vi "WaveGenerator_Sample_Program_NoDDL.vi"(0 "System no.":i32=1 min=1 step=1, 1 "Stop refnum":refnum<vi>, 2 "Affected axis":string="1", 3 "Selection":T1, 5 "error in":errorcluster, 6 "Sine Parameters:":T3={"Xo (Start)"=0, "SIN_P Parameters"={"C"=200.0, "A"=10.0, "O"=0.0}, "N (Length)"=500, "Append? (&)"=FALSE} {"N (Length)" min=0 max=1000 step=1; "SIN_P Parameters"."O" format="%.6f"; "SIN_P Parameters"."A" format="%.6f"; "SIN_P Parameters"."C" format="%.6f"}, 7 "Ramp Parameters:":T2={"Xo (Start)"=0, "RAMP Parameters"={"C"=200.0, "J"=0.0, "A"=8.0, "O"=0.0}, "N (Length)"=500, "Append? (&)"=FALSE} {"N (Length)" min=0 max=1000 step=1; "RAMP Parameters"."O" format="%.6f"; "RAMP Parameters"."A" format="%.6f"; "RAMP Parameters"."J" format="%.6f"; "RAMP Parameters"."C" format="%.6f"}, 8 "Start position":dbl format="%.6f") -> (14 "Waveform":dbl[][](graph) caption="Graph showing the commanded (green) and measured (white) waveform.", 19 "Error out":errorcluster)   [LabVIEW 2014, in "PiFOC.lvlib"]
doc: "This VI demonstrates how to use the wave generator command VIs. It first moves the affected axis to a given start position. Then it runs in a loop, giving the user the options to write sine wave curve segments or ramps into the controllers wave buffer. Wave storage data points are limited to 1000 points to keep transfer times low. The segment length of one waveform - which normally defines the frequency - is predefined as 500 points in this example. Depending on the value of Append? (&), either the old buffer data is overwritten or the new wave will be appended to memory. Please take into account that you can append at most two waveforms since buffer size is limited to 1000 points as mentioned above. \n\nAdjust the following controls to modify the shape of the waveforms.\nN (Length): Waveform (i.e. the points to be modified) goes from 1 to Length. Datapoints from Length to 500 are filled with value of last wave point.\nXo (Start): Position where the first point of the waveform is located. \nC: Center point of the wave. If C = Length/2 then the wave is symmetrical.\nA: Amplitude of the waveform. F(x) = A*sin(x) + O\nO: Offset of the waveform. F(x) = A*sin(x) + O\nJ: Jerk. Means curvature in the transition to or from standstill.\n\nYou have to stop generator output prior to restarting it with a different parameter set. The Start Gen. and Stop Gen. buttons will enable or disable the wave generator output by sending \"WGO 0\" or \"WGO 1\" for the affected axis. The red Stop button stops the wave generator output on the specified axis and finishes the loop. Please respect the delays that occur while the controller is processing your commands. This is indicated by the \"Busy?\" indicator. See manual for further details. \n\nIn case of an error a button Clear Error will appear and the control buttons above will be disabled. Pressing this button will clear the error status and enable the control buttons again.\n\nSee User Manual for details about the use of the wave generator.\n\nRun XXXX_Configuration_Setup (with XXXX being the product number of your PI controller) prior to running this VI.\n\nValid for: E-709"
uses:
  PiFOC.lvlib
panel:
  in  "Wave Table":string="1"
  out "Gen. running?":bool
  in  "Clear Error":bool
  out "Busy?":bool
  out "Controller error":bool
  in  "Stop":bool
  # "Wave generator sample program without DDL functionality"
  # "This VI demonstrates how to use the wave generator command VIs. It first moves the affected axis to a given start position. Then it runs in a loop, giving the\nuser the options to write sine wave curve segments or ramps into the controllers wave buffer. Wave storage data points are limited to 1000 points\nto keep transfer times low. The segment length of one waveform is predefined as 500 points in this example. Depending on the value of Append? (&), either\nthe old buffer data is overwritten or the new wave will be appended to memory. You have to stop generator output prior to restarting it with a different\nparameter set. The Start Gen. and Stop Gen. buttons will enable or disable the wave generator output by sending \"WGO 0\" or \"WGO 1\" for the affected axis. \nThe red Stop button stops the wave generator output on the specified axis and finishes the loop. Please respect the delays that occur while the controller is \nprocessing your commands. This is indicated by the \"Busy?\" indicator. See manual for further details. \nRun XXXX_Configuration_Setup (with XXXX being the product number of your PI controller) prior to running this VI."
  # "Stop VI\nand wave\ngenerator\noutput"
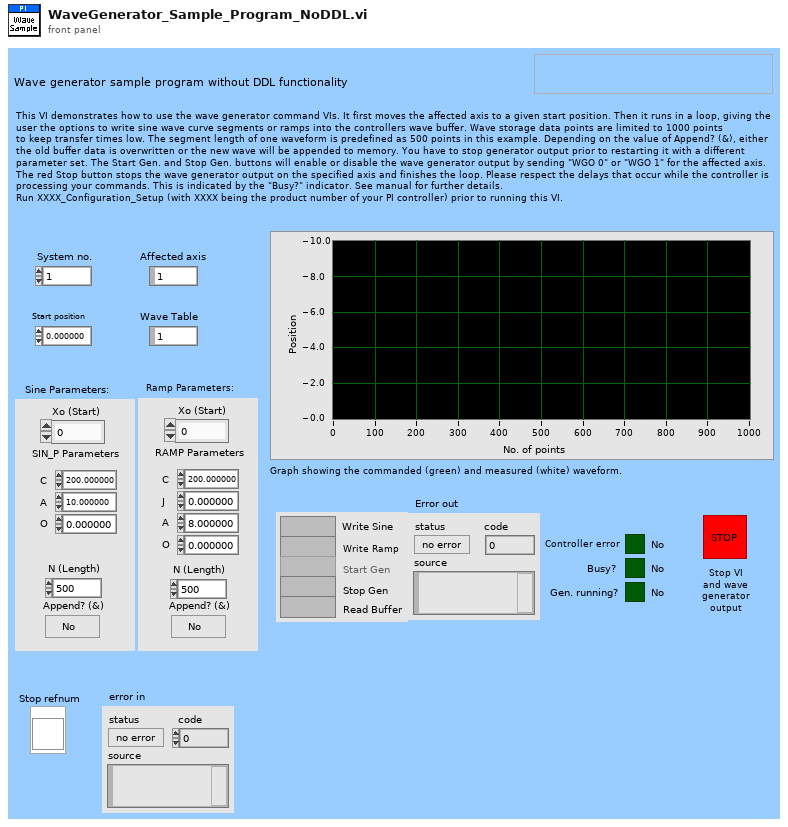
[diagram p1: front panel]
types:
  T1 = cluster{"Write Sine":bool, "Write Ramp":bool, "Start Gen":bool, "Stop Gen":bool, "Read Buffer":bool}
  T2 = cluster{"Xo (Start)":i32, "RAMP Parameters":cluster{"C":dbl, "J":dbl, "A":dbl, "O":dbl}, "N (Length)":i32, "Append? (&)":bool}
  T3 = cluster{"Xo (Start)":i32, "SIN_P Parameters":cluster{"C":dbl, "A":dbl, "O":dbl}, "N (Length)":i32, "Append? (&)":bool}
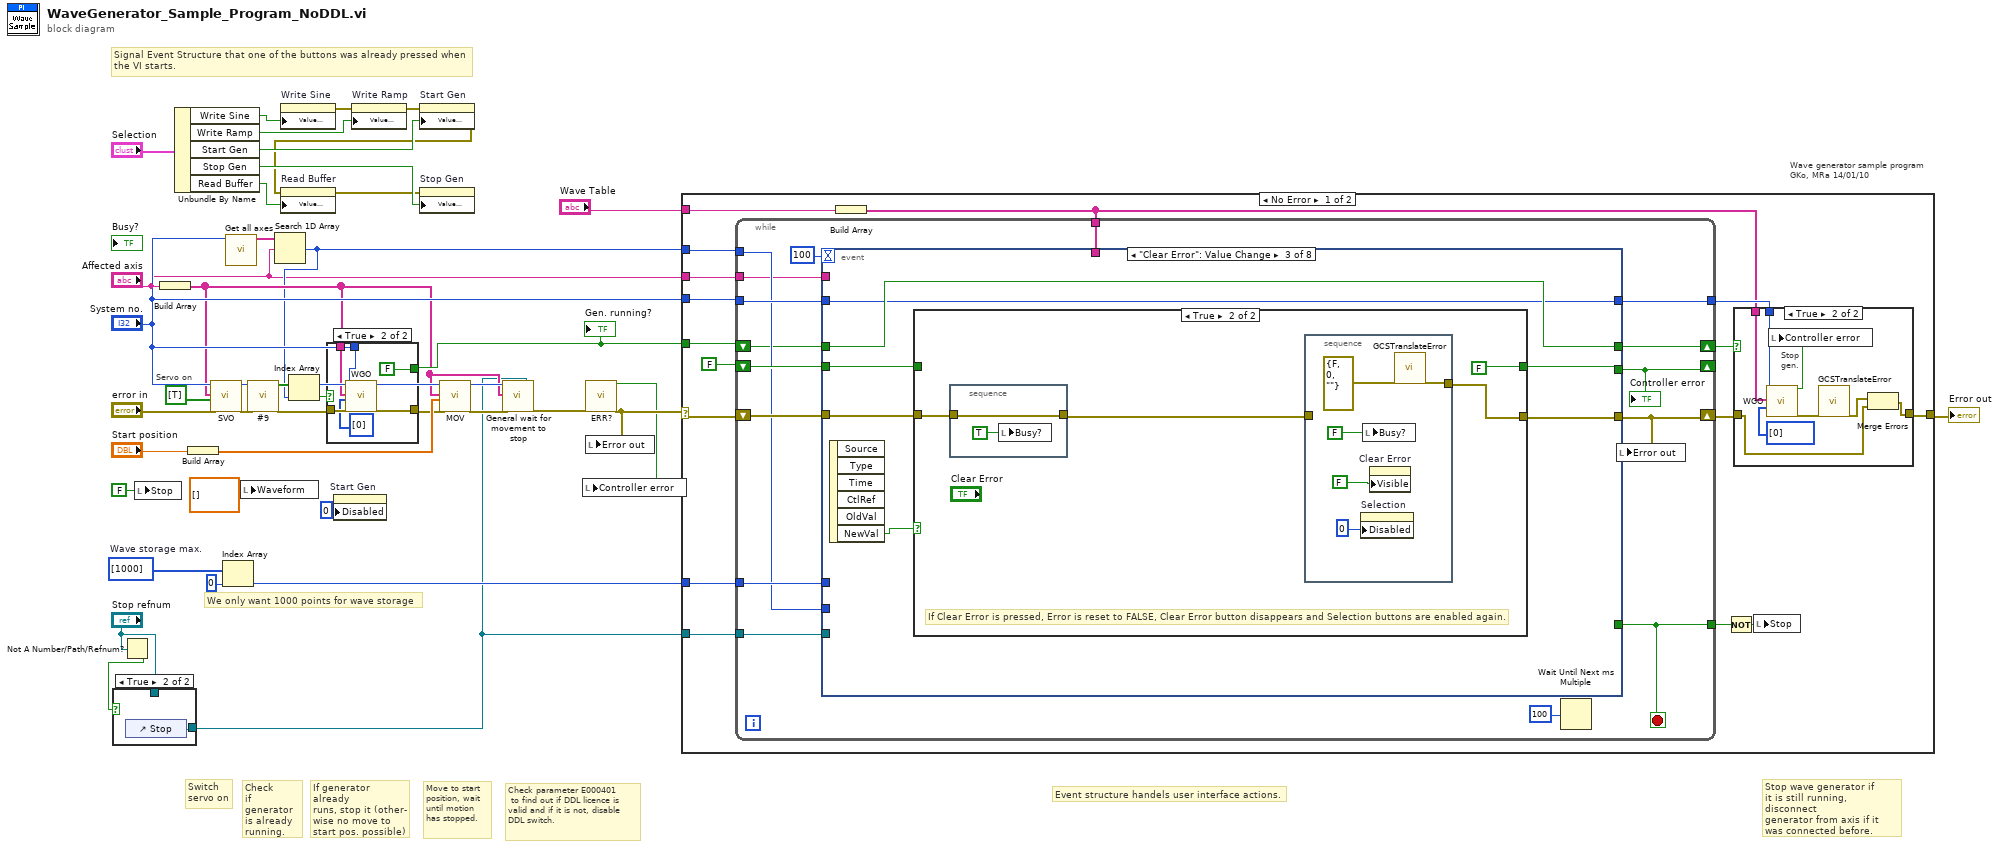
[diagram p0: block diagram]
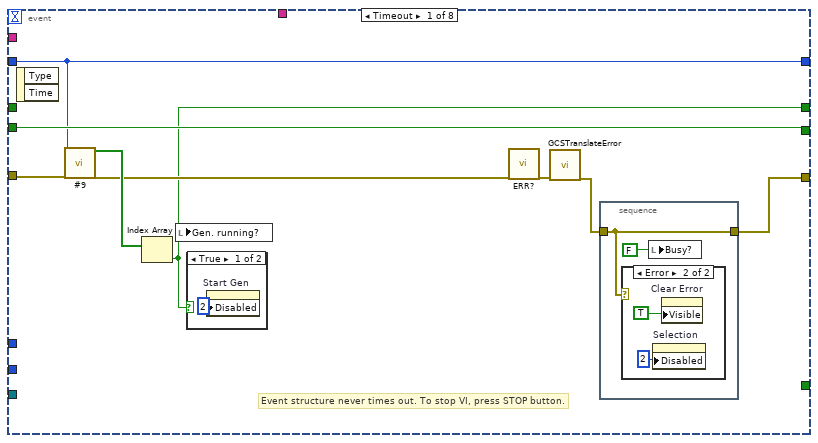
[diagram p5: hidden frame]
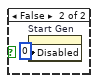
[diagram p7: hidden frame]
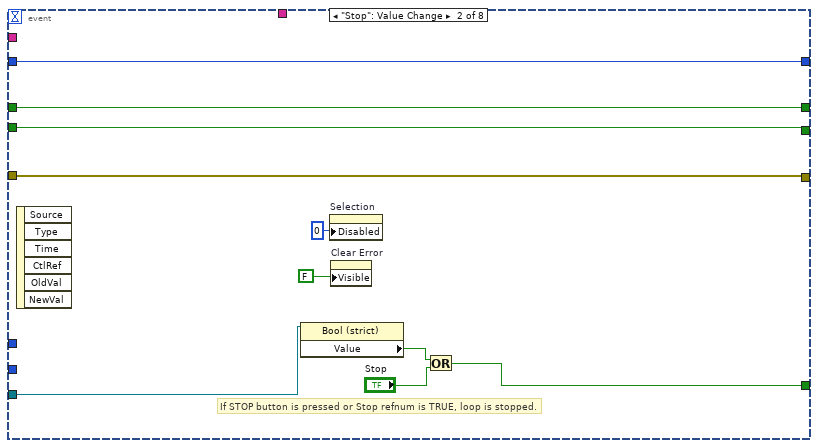
[diagram p8: hidden frame]
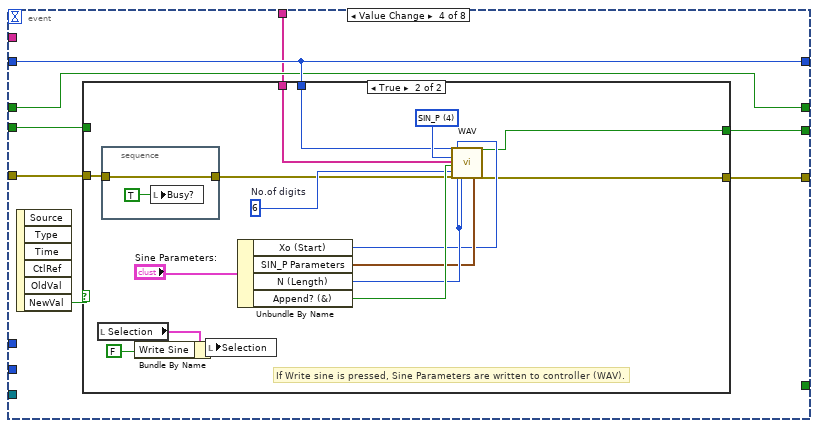
[diagram p10: hidden frame]
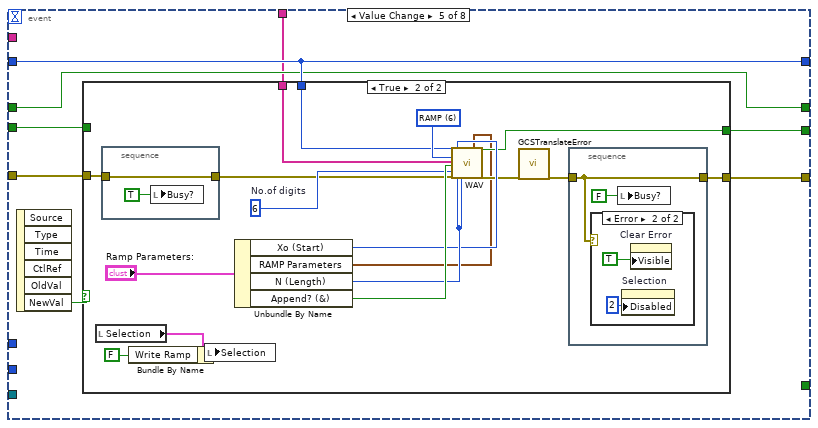
[diagram p12: hidden frame]
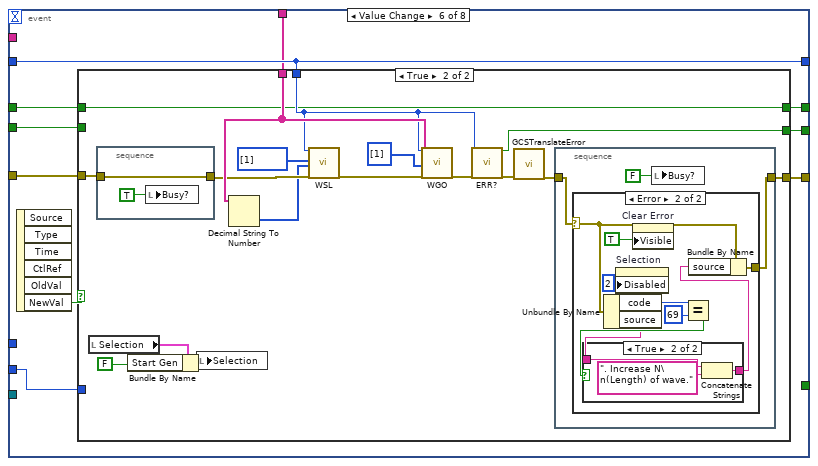
[diagram p15: hidden frame]
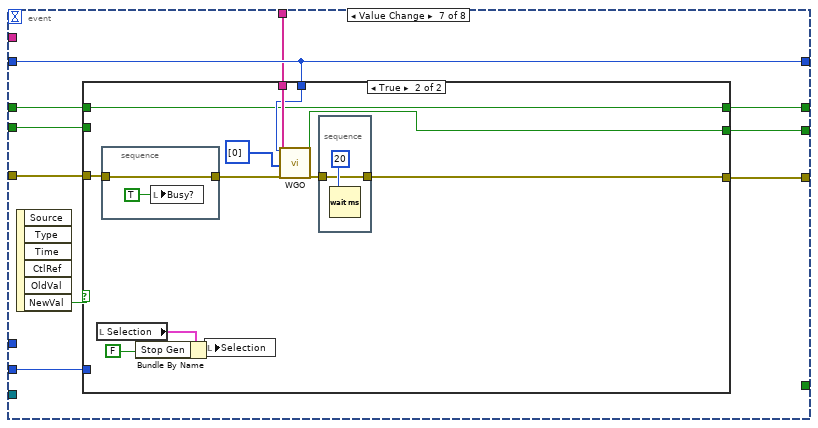
[diagram p19: hidden frame]
diagram:
  w37 = i32[] [1000]  # Wave storage max.
  # "Stop wave generator if\nit is still running, disconnect \ngenerator from axis if it\nwas connected before."
  # "Event structure handels user interface actions."
  # "Check parameter E000401\n to find out if DDL licence is\nvalid and if it is not, disable\nDDL switch."
  # "If generator already\nruns, stop it (other-\nwise no move to\nstart pos. possible)"
  # "Check\nif generator\nis already \nrunning."
  # "We only want 1000 points for wave storage"
  # "Switch\nservo on"
  # "Signal Event Structure that one of the buttons was already pressed when\nthe VI starts."
  # "Servo on"
  # "Move to start\nposition, wait\nuntil motion\nhas stopped."
  # "Wave generator sample program\nGKo, MRa 14/01/10"
  n1 = Not A Number/Path/Refnum?(number/path/refnum="Stop refnum") -> (NaN/Path/Refnum?=w33:bool)
  n2 = case shown="True" w33 {
    tunnel: [w41 w42] -> w9
    tunnel: "Stop refnum" -> [w41 _]
    frame False {
    }
    frame True {
      n3 = control-ref of="Stop"() -> (w42:refnum<vi>)
    }
  }
  n4 = local write "Stop"(FALSE ("Controller error")) -> ()
  n5 = Build Array("Affected axis") -> (w17:string[])
  n6 = Unbundle By Name("Selection") -> ("Write Sine"=w14:bool, "Write Ramp"=w13:bool, "Start Gen"=w12:bool, "Stop Gen"=w11:bool, "Read Buffer"=w10:bool)
  n7 = Build Array("Start position") -> (w34:dbl[])
  n8 = call "SVO.vi"("System no."="System no.", "Axes to command"=w17, "Servo mode"=bool[] [TRUE], "error in"="error in") -> ("error out"=w28:errorcluster)  [unwired: 1 in, 14 out]
  n9 = Index Array(array=w37, index=0 ("Index")) -> (element=w38:i32)
  n10 = call "Get all axes.vi"("System no."="System no.") -> ("Conn. Axes"=w29:string[])  [unwired: 18 out]
  n11 = local write "Waveform"(dbl[][] [] ("Waveform")) -> ()
  n12 = call "#9.vi"("System no."="System no.", "error in"=w28) -> ("WG running?"=w30:bool[], "error out"=w23:errorcluster)  [unwired: 16 out]
  n13 = Search 1D Array(1D array=w29, element="Affected axis") -> (index of element=w16:i32)  [unwired: 1 out]
  n14 = property on="Write Sine" class="Bool (strict)"("Value (Signaling)"=w14) -> (error out=w8:errorcluster)  [unwired: 2 in, 1 out]
  n15 = Index Array(array=w30, index=w16) -> (element=w24:bool)
  n16 = case shown="True" w24 {
    selector: w24 -> [w44 _]
    tunnel: w23 -> [w43 w50]
    tunnel: [w43 w49] -> w22
    tunnel: "System no." -> [_ w47]
    tunnel: w17 -> [_ w46]
    tunnel: [w44 FALSE] -> w21
    frame False {
    }
    frame True {
      n17 = call "WGO.vi"("System no."=w47, "Affected axes"=w46, "WGO Parameter"=i32[] [0], "error in"=w50) -> ("error out"=w49:errorcluster)  [unwired: 15 out]
    }
  }
  "Gen. running?" <- w21
  n18 = property on="Start Gen" class="Bool (strict)"("Disabled"=u8 0) -> ()  [unwired: 2 in, 2 out]
  n19 = property on="Write Ramp" class="Bool (strict)"(error in=w8, "Value (Signaling)"=w13) -> (error out=w7:errorcluster)  [unwired: 1 in, 1 out]
  n20 = property on="Start Gen" class="Bool (strict)"(error in=w7, "Value (Signaling)"=w12) -> (error out=w6:errorcluster)  [unwired: 1 in, 1 out]
  n21 = property on="Stop Gen" class="Bool (strict)"(error in=w6, "Value (Signaling)"=w11) -> (error out=w5:errorcluster)  [unwired: 1 in, 1 out]
  n22 = property on="Read Buffer" class="Bool (strict)"(error in=w5, "Value (Signaling)"=w10) -> ()  [unwired: 1 in, 2 out]
  n23 = call "MOV.vi"("System no."="System no.", "Axes to move"=w17, "Position values"=w34, "error in"=w22) -> ("error out"=w25:errorcluster)  [unwired: 1 in, 14 out]
  n24 = call "General wait for movement to stop.vi"("System no."="System no.", "Axes to wait for"=w17, "error in"=w25, "Stop refnum"=w9) -> ("error out"=w4:errorcluster)  [unwired: 4 in, 11 out]
  n25 = call "ERR?.vi"("error in"=w4) -> ("Controller error"=w3:bool, "error out"=w20:errorcluster)  [unwired: 1 in, 16 out]
  n26 = local write "Controller error"(w3) -> ()
  n27 = local write "Error out"(w20) -> ()
  n28 = case shown="No Error" w20 {
    selector: w20 -> [w61 w317]
    tunnel: "System no." -> [w66 _]
    tunnel: [w59 w316] -> w40
    tunnel: w38 -> [w62 _]
    tunnel: w16 -> [w60 _]
    tunnel: w21 -> [w58 _]
    tunnel: w9 -> [w54 _]
    tunnel: "Wave Table" -> [w53 _]
    tunnel: "Affected axis" -> [w52 _]
    frame No Error {
      n29 = Build Array(w53) -> (w51:string[])
      n30 = while {
        tunnel: w62 -> [w86]
        shift-left: w61 -> [w88]
        shift-right: [w87] -> w64
        tunnel: [w89] -> w65
        tunnel: w66 -> [w90]
        shift-right: [w84] -> _
        shift-left: FALSE ("Controller error") -> [w83]
        tunnel: w60 -> [w82]
        shift-right: [w80] -> w57
        shift-left: w58 -> [w81]
        tunnel: [w79] -> w56
        tunnel: w54 -> [w78]
        tunnel: w51 -> [w77]
        tunnel: w52 -> [w76]
        stop <- w79 stop-if-true
        n31 = event shown="[2] \"Clear Error\": Value Change" {
          selector: _ -> [_ _ _ _ _ _ _ _]
          dyn-events: _ -> [_ _ _ _ _ _ _ _]
          timeout: 100 -> [_ _ _ _ _ _ _ _]
          tunnel: w90 -> [w97 w114 w117 w139 w167 w203 w251 w279]
          tunnel: [w97 w114 w117 w139 w167 w203 w251 w279] -> w89
          tunnel: w88 -> [w98 w115 w119 w142 w170 w206 w255 w284]
          tunnel: [w93 w115 w120 w143 w171 w207 w256 w285] -> w87
          tunnel: w86 -> [_ _ _ _ _ _ _ w280]
          tunnel: [w100 w116 w121 w144 w172 w208 w257 w286] -> w84
          tunnel: w83 -> [w100 w116 w122 w140 w168 w204 w253 w282]
          tunnel: w82 -> [_ _ _ _ _ w200 w252 w281]
          tunnel: [_ w109 _ _ _ _ _ _] -> w79
          tunnel: w81 -> [_ w113 w118 w138 w166 w201 w249 w278]
          tunnel: [w92 w113 w118 w138 w166 w202 w250 w278] -> w80
          tunnel: w78 -> [_ w112 _ _ _ _ _ _]
          tunnel: w77 -> [_ _ _ w137 w165 w199 w248 _]
          tunnel: w76 -> [_ _ _ _ _ _ _ w277]
          event Timeout {
            # "Event structure never times out. To stop VI, press STOP button."
            n32 = event-data() -> ()  [unwired: 3 out]
            n33 = call "#9.vi"("System no."=w97, "error in"=w98) -> ("WG running?"=w99:bool[], "error out"=w94:errorcluster)  [unwired: 16 out]
            n34 = Index Array(array=w99) -> (element=w92:bool)  [unwired: 1 in]
            n35 = local write "Gen. running?"(w92) -> ()
            n36 = case shown="True" w92 {
              frame True {
                n37 = property on="Start Gen" class="Bool (strict)"("Disabled"=u8 2) -> ()  [unwired: 2 in, 2 out]
              }
              frame False {
                n38 = property on="Start Gen" class="Bool (strict)"("Disabled"=u8 0) -> ()  [unwired: 2 in, 2 out]
              }
            }
            n39 = call "ERR?.vi"("error in"=w94) -> ("error out"=w95:errorcluster)  [unwired: 1 in, 17 out]
            n40 = call "GCSTranslateError.vi"("error in"=w95) -> ("error out"=w96:errorcluster)  [unwired: 18 out]
            n41 = stacked-sequence {
              tunnel: w96 -> [w101]
              tunnel: [w101] -> w93
              frame #0 {
                n42 = case shown="Error" w101 {
                  frame No Error {
                  }
                  frame Error {
                    n43 = property on="Selection" class="Clust (strict)"("Disabled"=u8 2) -> ()  [unwired: 2 in, 2 out]
                    n44 = property on="Clear Error" class="Bool"("Visible"=TRUE) -> ()  [unwired: 2 in, 2 out]
                  }
                }
                n45 = local write "Busy?"(FALSE) -> ()
              }
            }
          }
          event "Stop": Value Change {
            # "If STOP button is pressed or Stop refnum is TRUE, loop is stopped."
            n46 = event-data() -> ()  [unwired: 7 out]
            n47 = property class="Bool (strict)"(reference=w112) -> ("Value"=w111:bool)  [unwired: 1 in, 2 out]
            n48 = property on="Selection" class="Clust (strict)"("Disabled"=u8 0) -> ()  [unwired: 2 in, 2 out]
            n49 = property on="Clear Error" class="Bool"("Visible"=FALSE) -> ()  [unwired: 2 in, 2 out]
            n50 = Or(x=w111, y="Stop") -> (x .or. y?=w109:bool)
          }
          event "Clear Error": Value Change {
            n51 = event-data() -> ("NewVal"=w123:bool)  [unwired: 6 out]
            n52 = case shown="True" w123 {
              tunnel: w122 -> [w125 _]
              tunnel: [w125 FALSE ("Controller error")] -> w121
              tunnel: [w124 w127] -> w120
              tunnel: w119 -> [w124 w128]
              frame False {
              }
              frame True {
                # "If Clear Error is pressed, Error is reset to FALSE, Clear Error button disappears and Selection buttons are enabled again."
                n53 = stacked-sequence {
                  tunnel: w128 -> [w135]
                  tunnel: [w135] -> w126
                  frame #0 {
                    n54 = local write "Busy?"(TRUE) -> ()
                  }
                }
                n55 = stacked-sequence {
                  tunnel: [w130] -> w127
                  tunnel: w126 -> [_]
                  frame #0 {
                    n56 = property on="Selection" class="Clust (strict)"("Disabled"=u8 0) -> ()  [unwired: 2 in, 2 out]
                    n57 = local write "Busy?"(FALSE) -> ()
                    n58 = property on="Clear Error" class="Bool"("Visible"=FALSE) -> ()  [unwired: 2 in, 2 out]
                    n59 = call "GCSTranslateError.vi"("error in"=errorcluster {"status"=FALSE, "code"=0, "source"=""} ("error IO")) -> ("error out"=w130:errorcluster)  [unwired: 18 out]
                  }
                }
              }
            }
          }
          event "Selection.Write Sine": Value Change {
            n60 = event-data() -> ("NewVal"=w141:bool)  [unwired: 6 out]
            n61 = case shown="True" w141 {
              tunnel: [w145 w155] -> w144
              tunnel: w139 -> [_ w150]
              tunnel: w137 -> [_ w149]
              tunnel: [w146 w147] -> w143
              tunnel: w142 -> [w146 w154]
              tunnel: w140 -> [w145 _]
              frame False {
              }
              frame True {
                w158 = i16 6  # No.of digits
                w157 = u16 4 items=["SIN", "POL", "TAN", "PNT", "SIN_P", "LIN", "RAMP"] ("Waveform")
                # "If Write sine is pressed, Sine Parameters are written to controller (WAV)."
                n62 = local read "Selection"() -> (w153:T1)
                n63 = stacked-sequence {
                  tunnel: w154 -> [w163]
                  tunnel: [w163] -> w148
                  frame #0 {
                    n64 = local write "Busy?"(TRUE) -> ()
                  }
                }
                n65 = Bundle By Name(cluster=w153, "Write Sine"=FALSE) -> (w152:T1)
                n66 = local write "Selection"(w152) -> ()
                n67 = Unbundle By Name("Sine Parameters:") -> ("Xo (Start)"=w159:i32, "SIN_P Parameters"=w160:cluster{"C":dbl, "A":dbl, "O":dbl}, "N (Length)"=w161:i32, "Append? (&)"=w162:bool)
                n68 = call "WAV.vi"("System no."=w150, "Waveform"=w157, "Affected axes"=w149, "Append? (&)"=w162, "No.of digits"=w158, "error in"=w148, "Xo"=w159, "N"=w161, "Segment length"=w161, "SIN_P Parameters"=w160) -> ("Controller error"=w155:bool, "error out"=w147:errorcluster)  [unwired: 9 in, 7 out]
              }
            }
          }
          event "Selection.Write Ramp": Value Change {
            n69 = event-data() -> ("NewVal"=w169:bool)  [unwired: 6 out]
            n70 = case shown="True" w169 {
              tunnel: [w173 w187] -> w172
              tunnel: w167 -> [_ w186]
              tunnel: w165 -> [_ w185]
              tunnel: [w174 w182] -> w171
              tunnel: w170 -> [w174 w181]
              tunnel: w168 -> [w173 _]
              frame False {
              }
              frame True {
                w189 = i16 6  # No.of digits
                w188 = u16 6 items=["SIN", "POL", "TAN", "PNT", "SIN_P", "LIN", "RAMP"] ("Waveform")
                n71 = local read "Selection"() -> (w177:T1)
                n72 = stacked-sequence {
                  tunnel: w181 -> [w193]
                  tunnel: [w193] -> w180
                  frame #0 {
                    n73 = local write "Busy?"(TRUE) -> ()
                  }
                }
                n74 = Bundle By Name(cluster=w177, "Write Ramp"=FALSE ("Write Sine")) -> (w176:T1)
                n75 = local write "Selection"(w176) -> ()
                n76 = Unbundle By Name("Ramp Parameters:") -> ("Xo (Start)"=w190:i32, "RAMP Parameters"=w178:cluster{"C":dbl, "J":dbl, "A":dbl, "O":dbl}, "N (Length)"=w191:i32, "Append? (&)"=w192:bool)
                n77 = call "WAV.vi"("System no."=w186, "Waveform"=w188, "Affected axes"=w185, "Append? (&)"=w192, "No.of digits"=w189, "error in"=w180, "Xo"=w190, "N"=w191, "Segment length"=w191, "RAMP Parameters"=w178) -> ("Controller error"=w187:bool, "error out"=w184:errorcluster)  [unwired: 9 in, 7 out]
                n78 = call "GCSTranslateError.vi"("error in"=w184) -> ("error out"=w183:errorcluster)  [unwired: 18 out]
                n79 = stacked-sequence {
                  tunnel: w183 -> [w195]
                  tunnel: [w195] -> w182
                  frame #0 {
                    n80 = case shown="Error" w195 {
                      frame No Error {
                      }
                      frame Error {
                        n81 = property on="Selection" class="Clust (strict)"("Disabled"=u8 2) -> ()  [unwired: 2 in, 2 out]
                        n82 = property on="Clear Error" class="Bool"("Visible"=TRUE) -> ()  [unwired: 2 in, 2 out]
                      }
                    }
                    n83 = local write "Busy?"(FALSE) -> ()
                  }
                }
              }
            }
          }
          event "Selection.Start Gen": Value Change {
            n84 = event-data() -> ("NewVal"=w205:bool)  [unwired: 6 out]
            n85 = case shown="True" w205 {
              tunnel: [w210 w222] -> w208
              tunnel: w203 -> [_ w214]
              tunnel: w199 -> [_ w221]
              tunnel: [w211 w227] -> w207
              tunnel: w206 -> [w211 w226]
              tunnel: w204 -> [w210 _]
              tunnel: [w209 w212] -> w202
              tunnel: w201 -> [w209 w212]
              tunnel: w200 -> [_ _]
              frame False {
              }
              frame True {
                n86 = local read "Selection"() -> (w220:T1)
                n87 = stacked-sequence {
                  tunnel: w226 -> [w229]
                  tunnel: [w229] -> w217
                  frame #0 {
                    n88 = local write "Busy?"(TRUE) -> ()
                  }
                }
                n89 = Bundle By Name(cluster=w220, "Start Gen"=FALSE ("Write Sine")) -> (w219:T1)
                n90 = local write "Selection"(w219) -> ()
                n91 = Decimal String To Number(string=w221) -> (number=w215:i32[])  [unwired: 3 out]
                n92 = call "WSL.vi"("System no."=w214, "Generator ID"=i32[] [1] ("WaveTableID"), "WaveTableID"=w215, "error in"=w217) -> ("error out"=w224:errorcluster)  [unwired: 15 out]
                n93 = call "WGO.vi"("System no."=w214, "Affected axes"=w221, "WGO Parameter"=i32[] [1], "error in"=w224) -> ("error out"=w213:errorcluster)  [unwired: 15 out]
                n94 = call "ERR?.vi"("System no."=w214, "error in"=w213) -> ("Controller error"=w222:bool, "error out"=w223:errorcluster)  [unwired: 16 out]
                n95 = call "GCSTranslateError.vi"("error in"=w223) -> ("error out"=w228:errorcluster)  [unwired: 18 out]
                n96 = stacked-sequence {
                  tunnel: w228 -> [w232]
                  tunnel: [w231] -> w227
                  frame #0 {
                    n97 = case shown="Error" w232 {
                      selector: w232 -> [w234 w239]
                      tunnel: [w234 w237] -> w231
                      frame No Error {
                      }
                      frame Error {
                        n98 = Unbundle By Name(w239) -> ("code"=w241:i32, "source"=w235:string)
                        n99 = property on="Selection" class="Clust (strict)"("Disabled"=u8 2) -> ()  [unwired: 2 in, 2 out]
                        n100 = property on="Clear Error" class="Bool"("Visible"=TRUE) -> ()  [unwired: 2 in, 2 out]
                        n101 = Equal?(x=w241, y=69) -> (x = y?=w236:bool)
                        n102 = case shown="True" w236 {
                          tunnel: [w244 w246] -> w238
                          tunnel: w235 -> [w244 w245]
                          frame False {
                          }
                          frame True {
                            n103 = Concatenate Strings(w245, ". Increase N\n(Length) of wave.") -> (w246:string)
                          }
                        }
                        n104 = Bundle By Name(cluster=w239, "source"=w238) -> (w237:errorcluster)
                      }
                    }
                    n105 = local write "Busy?"(FALSE) -> ()
                  }
                }
              }
            }
          }
          event "Selection.Stop Gen": Value Change {
            n106 = event-data() -> ("NewVal"=w254:bool)  [unwired: 6 out]
            n107 = case shown="True" w254 {
              tunnel: [w259 w261] -> w257
              tunnel: w251 -> [_ w267]
              tunnel: w248 -> [_ w270]
              tunnel: [w260 w263] -> w256
              tunnel: w255 -> [w260 w272]
              tunnel: w253 -> [w259 _]
              tunnel: w252 -> [_ _]
              tunnel: [w258 w262] -> w250
              tunnel: w249 -> [w258 w262]
              frame False {
              }
              frame True {
                n108 = local read "Selection"() -> (w266:T1)
                n109 = stacked-sequence {
                  tunnel: w272 -> [w275]
                  tunnel: [w275] -> w269
                  frame #0 {
                    n110 = local write "Busy?"(TRUE) -> ()
                  }
                }
                n111 = Bundle By Name(cluster=w266, "Stop Gen"=FALSE ("Write Sine")) -> (w265:T1)
                n112 = local write "Selection"(w265) -> ()
                n113 = call "WGO.vi"("System no."=w267, "Affected axes"=w270, "WGO Parameter"=i32[] [0], "error in"=w269) -> ("Controller error"=w261:bool, "error out"=w268:errorcluster)  [unwired: 14 out]
                n114 = stacked-sequence {
                  tunnel: w268 -> [w273]
                  tunnel: [w273] -> w263
                  frame #0 {
                    n115 = Wait (ms)(milliseconds to wait=u32 20) -> ()  [unwired: 1 out]
                  }
                }
              }
            }
          }
          event "Selection.Read Buffer": Value Change {
            n116 = event-data() -> ("NewVal"=w283:bool)  [unwired: 6 out]
            n117 = case shown="True" w283 {
              tunnel: [w287 w289] -> w286
              tunnel: w279 -> [_ w298]
              tunnel: [w288 w290] -> w285
              tunnel: w284 -> [w288 w313]
              tunnel: w282 -> [w287 _]
              tunnel: w281 -> [_ _]
              tunnel: w277 -> [_ w297]
              tunnel: w280 -> [_ w295]
              frame False {
              }
              frame True {
                w304 = 2 ("Numeric")
                w308 = 1 ("Numeric")
                # "Record and display values"
                n118 = stacked-sequence {
                  tunnel: w313 -> [w314]
                  tunnel: [w314] -> w299
                  frame #0 {
                    n119 = local write "Busy?"(TRUE) -> ()
                  }
                }
                n120 = call "DRC.vi"("System no."=w298, "Rec. table"=w308, "Rec. option"=w308, "error in"=w299, "Source ID"=w297) -> ("Controller error"=w303:bool, "error out"=w307:errorcluster)  [unwired: 1 in, 12 out]
                n121 = call "DRC.vi"("System no."=w298, "Rec. table"=w304, "Rec. option"=w304, "error in"=w307, "Source ID"=w297) -> ("Controller error"=w302:bool, "error out"=w291:errorcluster)  [unwired: 1 in, 12 out]
                n122 = call "WGR.vi"("System no."=w298, "error in"=w291) -> ("error out"=w300:errorcluster)  [unwired: 2 in, 15 out]
                n123 = call "DRR?.vi"("System no."=w298, "Rec. table IDs"=i32[] [1, 2], "error in"=w300, "Xo"=1, "N"=w295, "Nmax"=w295) -> ("Data"=w311:dbl[][], "error out"=w290:errorcluster)  [unwired: 2 in, 10 out]
                n124 = Index Array(array=w311, index (col) #1=0 ("Disabled Index (col)"), index (col) #2=1 ("Disabled Index (col)")) -> (element #1=w309:dbl[], element #2=w305:dbl[])  [unwired: 2 in]
                n125 = Build Array(w309, w305) -> (→"Waveform":dbl[][])
                n126 = Compound Arithmetic op=OR(w303, w302) -> (w289:bool)
                n127 = local read "Selection"() -> (w294:T1)
                n128 = Bundle By Name(cluster=w294, "Read Buffer"=FALSE ("Write Sine")) -> (w293:T1)
                n129 = local write "Selection"(w293) -> ()
              }
            }
          }
        }
        "Controller error" <- w84
        n130 = Wait Until Next ms Multiple(millisecond multiple=u32 100) -> ()  [unwired: 1 out]
        n131 = local write "Error out"(w87) -> ()
      }
      n132 = Not(x=w56) -> (.not. x?=w55:bool)
      n133 = case shown="True" w57 {
        tunnel: w65 -> [_ w73]
        tunnel: w64 -> [w67 w70]
        tunnel: [w67 w72] -> w59
        tunnel: w51 -> [_ w68]
        frame False {
        }
        frame True {
          # "Stop\ngen."
          n134 = call "WGO.vi"("System no."=w73, "Affected axes"=w68, "WGO Parameter"=i32[] [0] ("WGO \nParameter")) -> ("Controller error"=w74:bool, "error out"=w69:errorcluster)  [unwired: 1 in, 14 out]
          n135 = local write "Controller error"(w74) -> ()
          n136 = call "GCSTranslateError.vi"("error in"=w69) -> ("error out"=w71:errorcluster)  [unwired: 18 out]
          n137 = Merge Errors(w71, w70) -> (w72:errorcluster)
        }
      }
      n138 = local write "Stop"(w55) -> ()
    }
    frame Error {
      n139 = call "GCSTranslateError.vi"("error in"=w317) -> ("error out"=w316:errorcluster)  [unwired: 18 out]
    }
  }
  "Error out" <- w40
